vi "Cluster of M and N_UI.vi"(6 "ControlsIndicators":T1, 8 "error in (no error)":errorcluster, 9 "Threshold limits":refnum<vi>, 10 "Index":u8, 11 "Input ListBox Cluster":T7) -> (0 "error out":errorcluster, 3 "ListBox Cluster out":T7)   [LabVIEW 2019, in "ZenGage v3.0 UI.lvclass"]
doc: "This VI checks for entered value Range of connectors, Range for fail, Strict range for connectors and Strict range for fail. If entered values are <1, then it assigns default value 1 to controls."
uses:
  ZenGage v3.0 UI.lvclass
  Type Definitions/Edit tolerance settings/Rack Selection.ctl
  Type Definitions/Edit tolerance settings/Edit Tolerance Input.ctl
  <vilib>/Utility/miscctls.llb/LVPoint32TypeDef.ctl
  Type Definitions/General/Master sample references.ctl
  Type Definitions/Controls and Indicators/Select a part (combobox).ctl
  Type Definitions/Controls and Indicators/EDL control references.ctl
  Type Definitions/Controls and Indicators/Diagnostics control referencs.ctl
  Type Definitions/Controls and Indicators/Inspection control references.ctl
  Type Definitions/Controls and Indicators/General_Control references.ctl
  Type Definitions/Controls and Indicators/Controls and Indicators Cluster.ctl
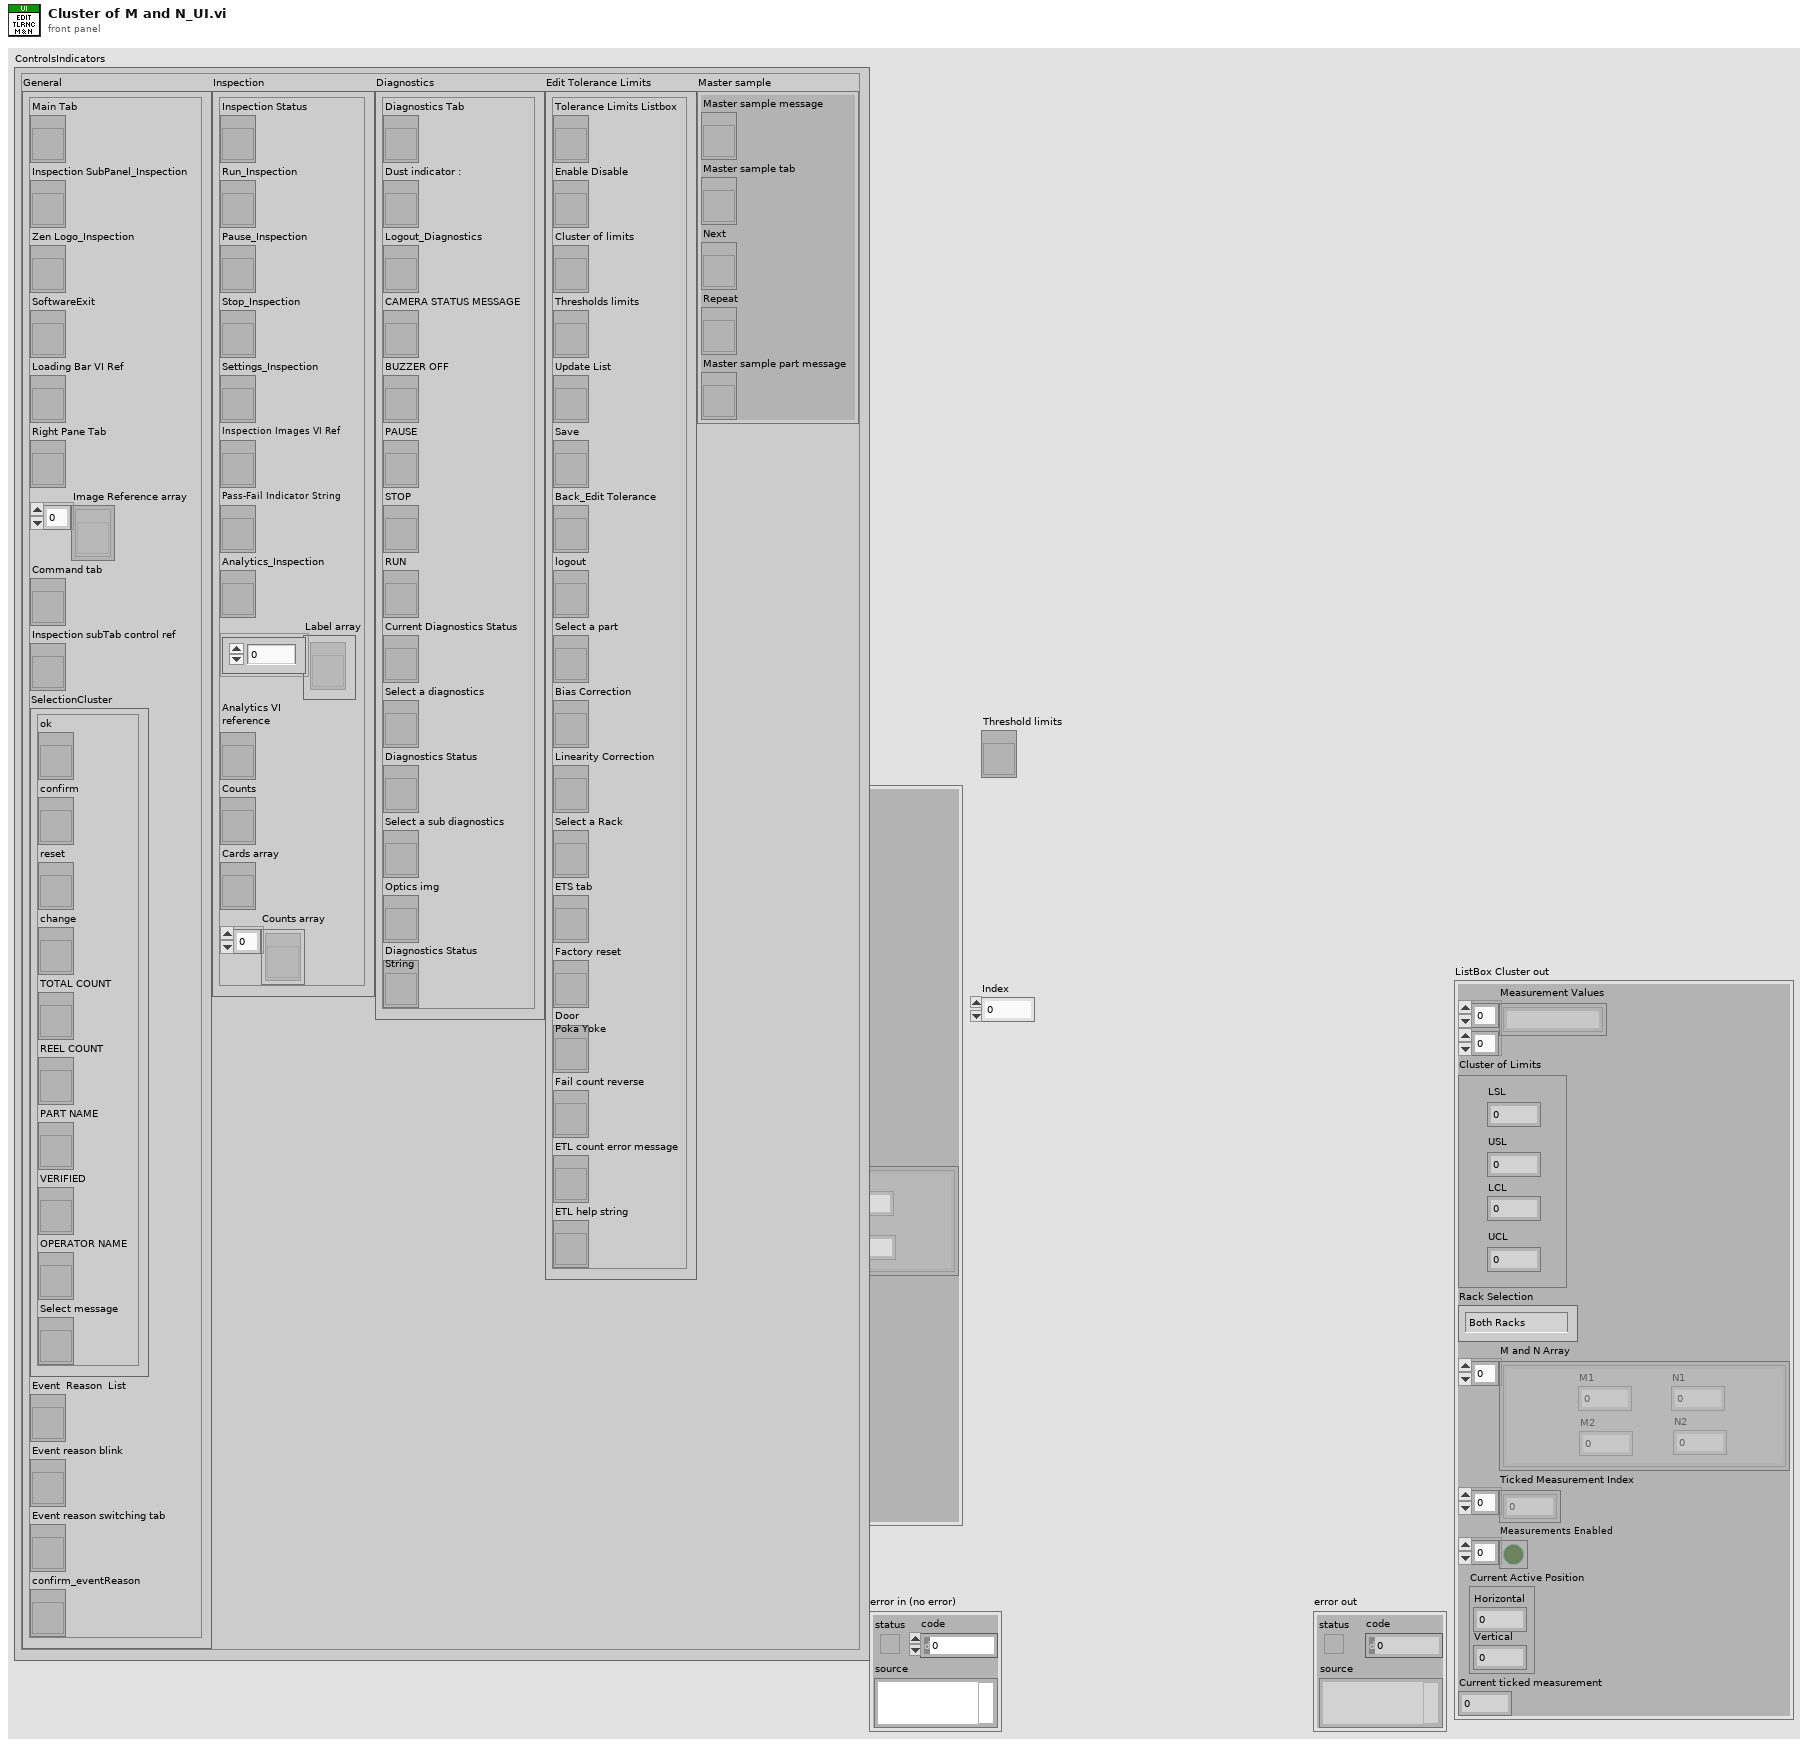
[diagram p1: front panel]
types:
  T1 = typedef "ZenGage v3.0 UI.lvclass/Controls and Indicators Cluster.ctl" = cluster{"General":T2, "Inspection":T3, "Diagnostics":T4, "Edit Tolerance Limits":T5, "Master sample":T6}
  T2 = typedef "ZenGage v3.0 UI.lvclass/General_Control references.ctl" = cluster{"Main Tab":refnum<vi>, "Inspection SubPanel_Inspection":refnum<vi>, "Zen Logo_Inspection":refnum<vi>, "SoftwareExit":refnum<vi>, "Loading Bar VI Ref":refnum<vi>, "Right Pane Tab":refnum<vi>, "Image Reference array":refnum<vi>[], "Command tab":refnum<vi>, "Inspection subTab control ref":refnum<vi>, "SelectionCluster":cluster{"ok":refnum<vi>, "confirm":refnum<vi>, "reset":refnum<vi>, "change":refnum<vi>, "TOTAL COUNT":refnum<vi>, "REEL COUNT":refnum<vi>, "PART NAME":refnum<vi>, "VERIFIED":refnum<vi>, "OPERATOR NAME":refnum<vi>, "Select message":refnum<vi>}, "Event  Reason  List":refnum<vi>, "Event reason blink":refnum<vi>, "Event reason switching tab":refnum<vi>, "confirm_eventReason":refnum<vi>}
  T3 = typedef "ZenGage v3.0 UI.lvclass/Inspection control references.ctl" = cluster{"Inspection Status":refnum<vi>, "Run_Inspection":refnum<vi>, "Pause_Inspection":refnum<vi>, "Stop_Inspection":refnum<vi>, "Settings_Inspection":refnum<vi>, "Inspection Images VI Ref":refnum<vi>, "Pass-Fail Indicator String":refnum<vi>, "Analytics_Inspection":refnum<vi>, "Label array":refnum<vi>[], "Analytics VI\nreference":refnum<vi>, "Counts":refnum<vi>, "Cards array":refnum<vi>, "Counts array":refnum<vi>[]}
  T4 = typedef "ZenGage v3.0 UI.lvclass/Diagnostics control referencs.ctl" = cluster{"Diagnostics Tab":refnum<vi>, "Dust indicator :":refnum<vi>, "Logout_Diagnostics":refnum<vi>, "CAMERA STATUS MESSAGE":refnum<vi>, "BUZZER OFF":refnum<vi>, "PAUSE":refnum<vi>, "STOP":refnum<vi>, "RUN":refnum<vi>, "Current Diagnostics Status":refnum<vi>, "Select a diagnostics":refnum<vi>, "Diagnostics Status":refnum<vi>, "Select a sub diagnostics":refnum<vi>, "Optics img":refnum<vi>, "Diagnostics Status\nString":refnum<vi>}
  T5 = typedef "ZenGage v3.0 UI.lvclass/EDL control references.ctl" = cluster{"Tolerance Limits Listbox":refnum<vi>, "Enable Disable":refnum<vi>, "Cluster of limits":refnum<vi>, "Thresholds limits":refnum<vi>, "Update List":refnum<vi>, "Save":refnum<vi>, "Back_Edit Tolerance":refnum<vi>, "logout":refnum<vi>, "Select a part":refnum<vi>, "Bias Correction":refnum<vi>, "Linearity Correction":refnum<vi>, "Select a Rack":refnum<vi>, "ETS tab":refnum<vi>, "Factory reset":refnum<vi>, "Door\nPoka Yoke":refnum<vi>, "Fail count reverse":refnum<vi>, "ETL count error message":refnum<vi>, "ETL help string":refnum<vi>}
  T6 = typedef "Master sample references.ctl" = cluster{"Master sample message":refnum<vi>, "Master sample tab":refnum<vi>, "Next":refnum<vi>, "Repeat":refnum<vi>, "Master sample part message":refnum<vi>}
  T7 = typedef "ZenGage v3.0 UI.lvclass/Edit Tolerance Input.ctl" = cluster{"Measurement Values":string[][], "Cluster of Limits":cluster{"LSL":dbl, "USL":dbl, "LCL":dbl, "UCL":dbl}, "Rack Selection":T8, "M and N Array":cluster{"M1":u64, "M2":u64, "N1":u64, "N2":u64}[], "Ticked Measurement Index":u32[], "Measurements Enabled":bool[], "Current Active Position":T9, "Current ticked measurement":dbl}
  T8 = typedef "ZenGage v3.0 UI.lvclass/Rack Selection.ctl" = enum16{"Both Racks", "Rack 2", "Rack 1"}
  T9 = typedef "LVPoint32TypeDef.ctl" = cluster{"Horizontal":i32, "Vertical":i32}
  T10 = enum8{"Enabled", "Disabled", "Disabled and Grayed Out"}
  T11 = cluster{"M1":u64, "M2":u64, "N1":u64, "N2":u64}[]
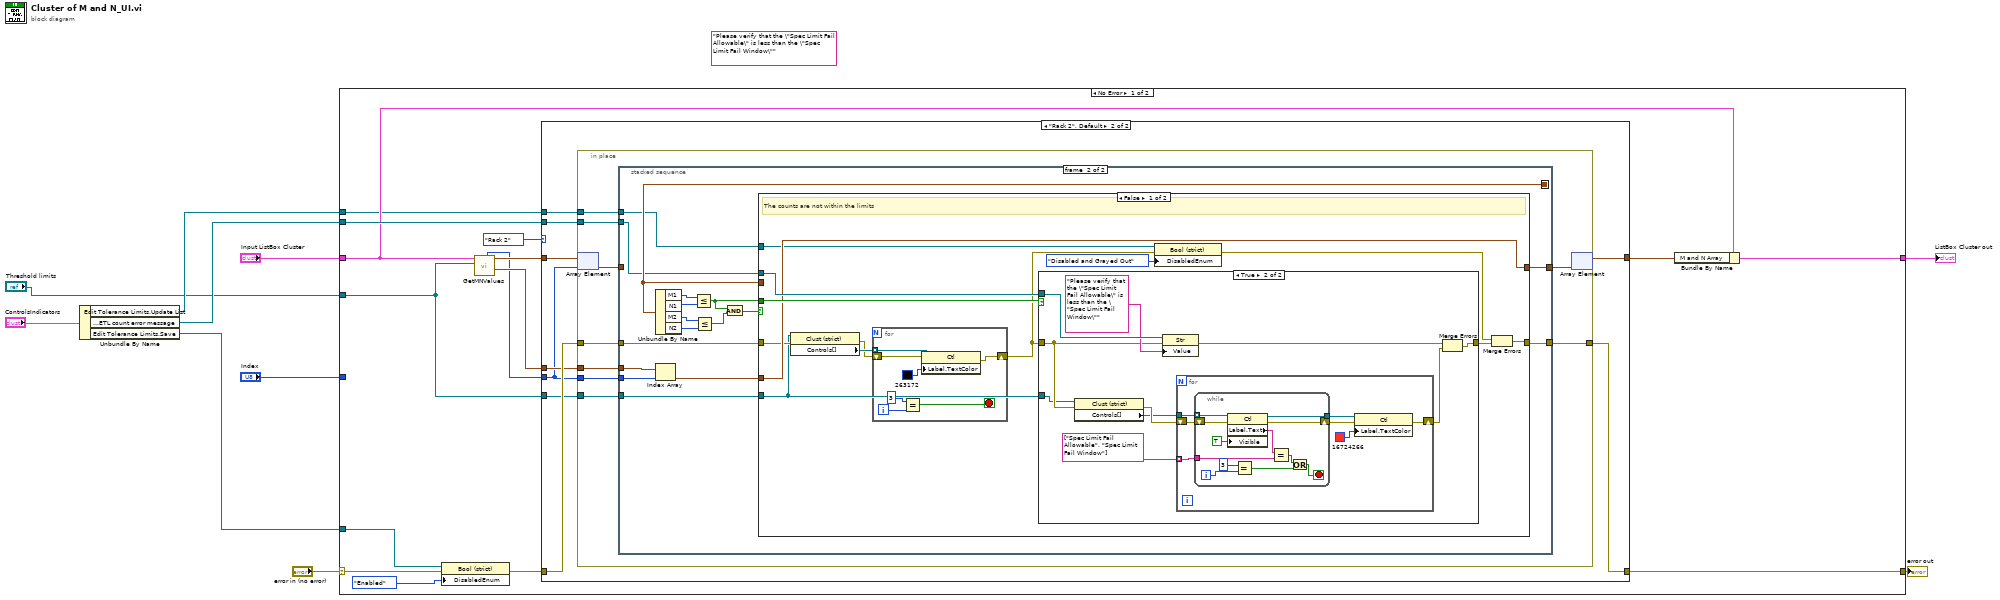
[diagram p0: block diagram]
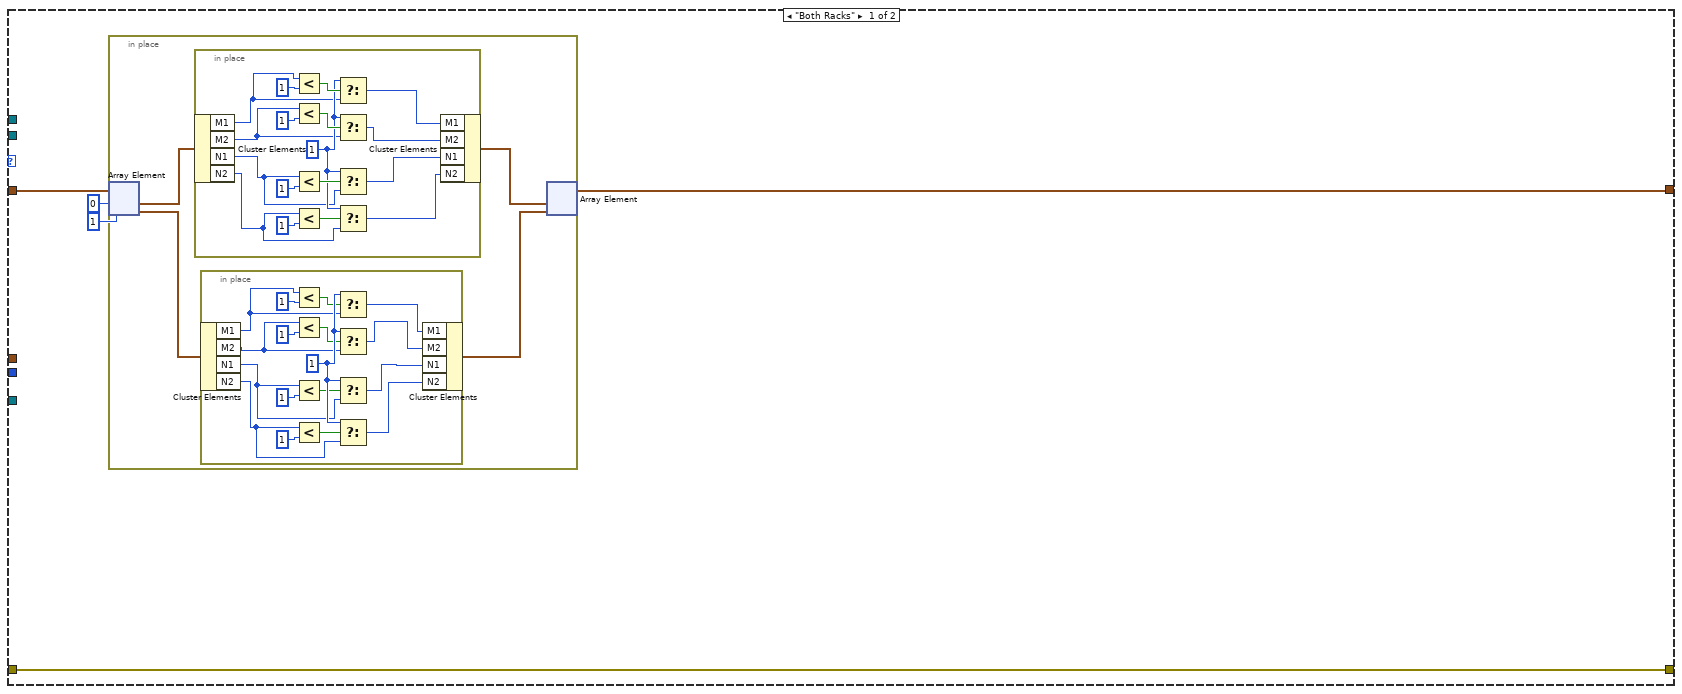
[diagram p2: hidden frame]
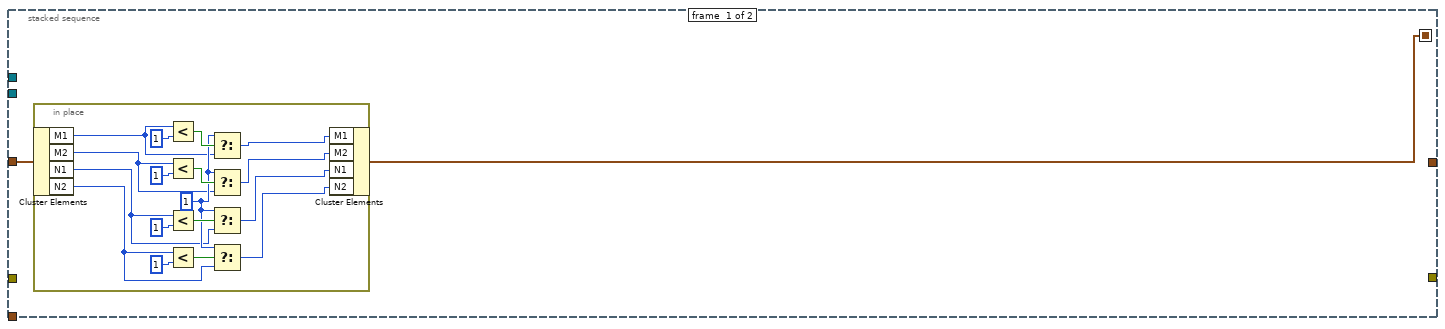
[diagram p3: hidden frame]
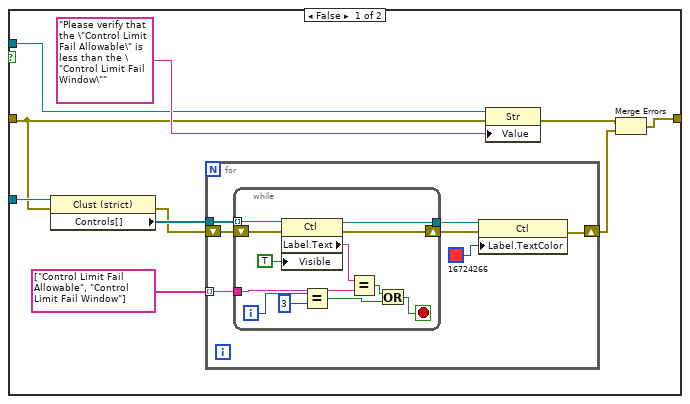
[diagram p4: hidden frame]
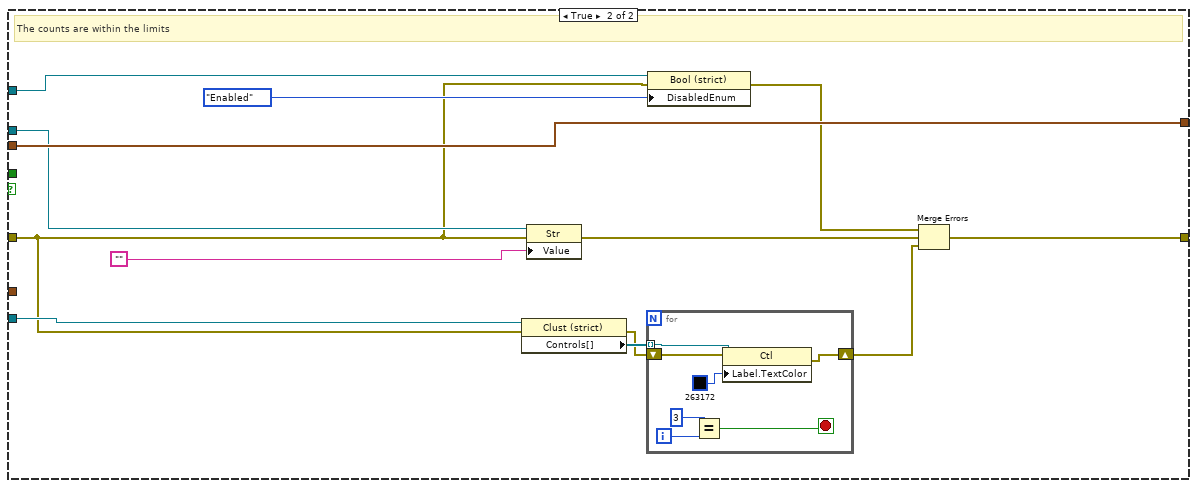
[diagram p5: hidden frame]
diagram:
  (unwired) "Please verify that the \"Spec Limit Fail Allowable\" is less than the \"Spec Limit Fail Window\"" ("Value")
  n1 = Unbundle By Name("ControlsIndicators") -> ("Edit Tolerance Limits.Update List"=w2:refnum<vi>, "Edit Tolerance Limits.ETL count error message"=w4:refnum<vi>, "Edit Tolerance Limits.Save"=w3:refnum<vi>)
  n2 = case shown="No Error" "error in (no error)" {
    selector: "error in (no error)" -> [w18 w222]
    tunnel: [w21 w222] -> w9
    tunnel: [w25 w221] -> w7
    tunnel: "Input ListBox Cluster" -> [w19 w221]
    tunnel: "Index" -> [_ _]
    tunnel: "Threshold limits" -> [w13 _]
    tunnel: w4 -> [w22 _]
    tunnel: w3 -> [w15 _]
    tunnel: w2 -> [w14 _]
    frame No Error {
      n3 = property class="Bool (strict)"(reference=w15, error in=w18, "DisabledEnum"=T10."Enabled" ("Disabled")) -> (error out=w17:errorcluster)  [unwired: 1 out]
      n4 = call "GetMNValues.vi"("Threshold limits"=w13, "Input ListBox Cluster in"=w19) -> ("M and N Array unchanged"=w20:T11, "MN Array changed"=w24:T11, "Last ticked measurement"=w11:u32)  [unwired: 5 in, 2 out]
      n5 = case shown="\"Rack 2\", Default" Rack_Selection."Rack 2" ("Rack Selection") {
        tunnel: w24 -> [w30 w77]
        tunnel: [w27 w76] -> w23
        tunnel: w11 -> [_ w71]
        tunnel: w17 -> [w26 w75]
        tunnel: w22 -> [_ w74]
        tunnel: [w26 w73] -> w21
        tunnel: w20 -> [_ w72]
        tunnel: w13 -> [_ w70]
        tunnel: w14 -> [_ w69]
        frame "Both Racks" {
          n6 = in-place {
            n7 = in-place-array #1(w30, 0, 1) -> (w34:cluster{"M1":u64, "M2":u64, "N1":u64, "N2":u64}, w33:cluster{"M1":u64, "M2":u64, "N1":u64, "N2":u64})
            n8 = in-place {
              w43 = u64 1 ("y")
              n9 = in-place-cluster #2(w34) -> ("M1"=w42:u64, "M2"=w41:u64, "N1"=w40:u64, "N2"=w39:u64)
              n10 = Less?(x=w42, y=u64 1) -> (x < y?=w47:bool)
              n11 = Less?(x=w41, y=u64 1) -> (x < y?=w46:bool)
              n12 = Less?(x=w40, y=u64 1) -> (x < y?=w45:bool)
              n13 = Less?(x=w39, y=u64 1) -> (x < y?=w44:bool)
              n14 = Select(t=w43, s=w47, f=w42) -> (s? t:f=w38:u64)
              n15 = Select(t=w43, s=w46, f=w41) -> (s? t:f=w37:u64)
              n16 = Select(t=w43, s=w45, f=w40) -> (s? t:f=w36:u64)
              n17 = Select(t=w43, s=w44, f=w39) -> (s? t:f=w35:u64)
              n18 = in-place-cluster #2("M1"=w38, "M2"=w37, "N1"=w36, "N2"=w35) -> (w31:cluster{"M1":u64, "M2":u64, "N1":u64, "N2":u64})
            }
            n19 = in-place {
              w68 = u64 1 ("y")
              n20 = in-place-cluster #3(w33) -> ("M1"=w59:u64, "M2"=w58:u64, "N1"=w57:u64, "N2"=w56:u64)
              n21 = Less?(x=w59, y=u64 1) -> (x < y?=w64:bool)
              n22 = Less?(x=w58, y=u64 1) -> (x < y?=w65:bool)
              n23 = Less?(x=w57, y=u64 1) -> (x < y?=w66:bool)
              n24 = Less?(x=w56, y=u64 1) -> (x < y?=w67:bool)
              n25 = Select(t=w68, s=w64, f=w59) -> (s? t:f=w55:u64)
              n26 = Select(t=w68, s=w65, f=w58) -> (s? t:f=w54:u64)
              n27 = Select(t=w68, s=w66, f=w57) -> (s? t:f=w53:u64)
              n28 = Select(t=w68, s=w67, f=w56) -> (s? t:f=w52:u64)
              n29 = in-place-cluster #3("M1"=w55, "M2"=w54, "N1"=w53, "N2"=w52) -> (w32:cluster{"M1":u64, "M2":u64, "N1":u64, "N2":u64})
            }
            n30 = in-place-array #1(w31, w32) -> (w27:T11)  [unwired: 2 out]
          }
        }
        frame "Rack 2", Default {
          n31 = in-place {
            in-place-border: w75 -> [w84]
            in-place-border: w74 -> [w83]
            in-place-border: [w82] -> w73
            in-place-border: w72 -> [w81]
            in-place-border: w71 -> [w80]
            in-place-border: w70 -> [w79]
            in-place-border: w69 -> [w78]
            n32 = in-place-array #4(w77, w71) -> (w86:cluster{"M1":u64, "M2":u64, "N1":u64, "N2":u64})
            n33 = stacked-sequence {
              seq-local: [w87 _] -> [_ w116]
              tunnel: w86 -> [w88 _]
              tunnel: [_ w115] -> w85
              tunnel: w84 -> [_ w113]
              tunnel: w83 -> [_ w112]
              tunnel: [_ w111] -> w82
              tunnel: w81 -> [_ w110]
              tunnel: w80 -> [_ w109]
              tunnel: w79 -> [_ w107]
              tunnel: w78 -> [_ w106]
              frame #0 {
                n34 = in-place {
                  w97 = u64 1 ("y")
                  n35 = in-place-cluster #5(w88) -> ("M1"=w96:u64, "M2"=w95:u64, "N1"=w94:u64, "N2"=w93:u64)
                  n36 = Less?(x=w96, y=u64 1) -> (x < y?=w101:bool)
                  n37 = Less?(x=w95, y=u64 1) -> (x < y?=w100:bool)
                  n38 = Less?(x=w94, y=u64 1) -> (x < y?=w99:bool)
                  n39 = Less?(x=w93, y=u64 1) -> (x < y?=w98:bool)
                  n40 = Select(t=w97, s=w101, f=w96) -> (s? t:f=w92:u64)
                  n41 = Select(t=w97, s=w100, f=w95) -> (s? t:f=w91:u64)
                  n42 = Select(t=w97, s=w99, f=w94) -> (s? t:f=w90:u64)
                  n43 = Select(t=w97, s=w98, f=w93) -> (s? t:f=w89:u64)
                  n44 = in-place-cluster #5("M1"=w92, "M2"=w91, "N1"=w90, "N2"=w89) -> (w87:cluster{"M1":u64, "M2":u64, "N1":u64, "N2":u64})
                }
              }
              frame #1 {
                n45 = Unbundle By Name(w116) -> ("M1"=w122:u64, "N1"=w121:u64, "M2"=w120:u64, "N2"=w119:u64)
                n46 = Index Array(array=w110, index=w109) -> (element=w108:cluster{"M1":u64, "M2":u64, "N1":u64, "N2":u64})
                n47 = Less Or Equal?(x=w122, y=w121) -> (x <= y?=w114:bool)
                n48 = Less Or Equal?(x=w120, y=w119) -> (x <= y?=w118:bool)
                n49 = And(x=w114, y=w118) -> (x .and. y?=w117:bool)
                n50 = case shown="False" w117 {
                  tunnel: w116 -> [_ w213]
                  tunnel: [w133 w213] -> w115
                  tunnel: w114 -> [w135 _]
                  tunnel: w113 -> [w125 w203]
                  tunnel: w112 -> [w134 w209]
                  tunnel: [w129 w206] -> w111
                  tunnel: w108 -> [w133 _]
                  tunnel: w107 -> [w124 w212]
                  tunnel: w106 -> [w132 w202]
                  frame False {
                    # "The counts are not within the limits"
                    n51 = property class="Clust (strict)"(reference=w124, error in=w125) -> (error out=w126:errorcluster, "Controls[]"=w127:refnum<vi>[])  [unwired: 1 out]
                    n52 = for {
                      tunnel: w127 -> [w140] mode=indexing
                      shift-right: [w139] -> w123
                      shift-left: w126 -> [w141]
                      i -> [w138]
                      stop <- w136 stop-if-true
                      n53 = Equal?(x=3, y=w138) -> (x = y?=w136:bool)
                      n54 = property class="Ctl"(reference=w140, error in=w141, "Label.TextColor"=u32 263172) -> (error out=w139:errorcluster)  [unwired: 1 out]
                    }
                    n55 = case shown="True" w135 {
                      tunnel: w123 -> [w149 w176]
                      tunnel: w134 -> [w151 w181]
                      tunnel: [w143 w172] -> w130
                      tunnel: w124 -> [w150 w175]
                      frame False {
                        n56 = property class="Clust (strict)"(reference=w150, error in=w149) -> (error out=w147:errorcluster, "Controls[]"=w148:refnum<vi>[])  [unwired: 1 out]
                        n57 = for {
                          tunnel: w148 -> [w159]
                          shift-right: [w155] -> w145
                          shift-left: w147 -> [w158]
                          tunnel: string[] ["Control Limit Fail Allowable", "Control Limit Fail Window"] -> [w157] mode=indexing
                          n58 = while {
                            tunnel: w159 -> [w171] mode=indexing
                            shift-right: [w169] -> w156
                            shift-left: w158 -> [w170]
                            tunnel: w157 -> [w167]
                            tunnel: [w166] -> w154
                            i -> [w163]
                            stop <- w161 stop-if-true
                            n59 = property class="Ctl"(reference=w171, error in=w170, "Visible"=TRUE) -> (reference out=w166:refnum<vi>, error out=w169:errorcluster, "Label.Text"=w168:string)
                            n60 = Equal?(x=w163, y=3) -> (x = y?=w164:bool)
                            n61 = Equal?(x=w168, y=w167) -> (x = y?=w165:bool)
                            n62 = Or(x=w165, y=w164) -> (x .or. y?=w161:bool)
                          }
                          n63 = property class="Ctl"(reference=w154, error in=w156, "Label.TextColor"=u32 16724266) -> (error out=w155:errorcluster)  [unwired: 1 out]
                        }
                        n64 = property class="Str"(reference=w151, error in=w149, "Value"="Please verify that the \"Control Limit Fail Allowable\" is less than the \"Control Limit Fail Window\"") -> (error out=w144:errorcluster)  [unwired: 1 out]
                        n65 = Merge Errors(w144, w145) -> (w143:errorcluster)
                      }
                      frame True {
                        n66 = property class="Clust (strict)"(reference=w175, error in=w176) -> (error out=w178:errorcluster, "Controls[]"=w177:refnum<vi>[])  [unwired: 1 out]
                        n67 = property class="Str"(reference=w181, error in=w176, "Value"="Please verify that the \"Spec Limit Fail Allowable\" is less than the \"Spec Limit Fail Window\"") -> (error out=w174:errorcluster)  [unwired: 1 out]
                        n68 = for {
                          tunnel: w177 -> [w188]
                          shift-right: [w184] -> w173
                          shift-left: w178 -> [w187]
                          tunnel: string[] ["Spec Limit Fail Allowable", "Spec Limit Fail Window"] -> [w186] mode=indexing
                          n69 = while {
                            tunnel: w188 -> [w200] mode=indexing
                            shift-right: [w198] -> w185
                            shift-left: w187 -> [w199]
                            tunnel: w186 -> [w196]
                            tunnel: [w195] -> w183
                            i -> [w194]
                            stop <- w190 stop-if-true
                            n70 = property class="Ctl"(reference=w200, error in=w199, "Visible"=TRUE) -> (reference out=w195:refnum<vi>, error out=w198:errorcluster, "Label.Text"=w197:string)
                            n71 = Equal?(x=3, y=w194) -> (x = y?=w192:bool)
                            n72 = Equal?(x=w197, y=w196) -> (x = y?=w191:bool)
                            n73 = Or(x=w191, y=w192) -> (x .or. y?=w190:bool)
                          }
                          n74 = property class="Ctl"(reference=w183, error in=w185, "Label.TextColor"=u32 16724266) -> (error out=w184:errorcluster)  [unwired: 1 out]
                        }
                        n75 = Merge Errors(w174, w173) -> (w172:errorcluster)
                      }
                    }
                    n76 = property class="Bool (strict)"(reference=w132, error in=w123, "DisabledEnum"=T10."Disabled and Grayed Out" ("Disabled")) -> (error out=w128:errorcluster)  [unwired: 1 out]
                    n77 = Merge Errors(w128, w130) -> (w129:errorcluster)
                  }
                  frame True {
                    # "The counts are within the limits"
                    n78 = property class="Clust (strict)"(reference=w212, error in=w203) -> (error out=w210:errorcluster, "Controls[]"=w211:refnum<vi>[])  [unwired: 1 out]
                    n79 = property class="Str"(reference=w209, error in=w203, "Value"="") -> (error out=w208:errorcluster)  [unwired: 1 out]
                    n80 = for {
                      tunnel: w211 -> [w218] mode=indexing
                      shift-right: [w217] -> w207
                      shift-left: w210 -> [w219]
                      i -> [w216]
                      stop <- w214 stop-if-true
                      n81 = Equal?(x=3, y=w216) -> (x = y?=w214:bool)
                      n82 = property class="Ctl"(reference=w218, error in=w219, "Label.TextColor"=u32 263172) -> (error out=w217:errorcluster)  [unwired: 1 out]
                    }
                    n83 = property class="Bool (strict)"(reference=w202, error in=w203, "DisabledEnum"=T10."Enabled" ("Disabled")) -> (error out=w201:errorcluster)  [unwired: 1 out]
                    n84 = Merge Errors(w201, w208, w207) -> (w206:errorcluster)
                  }
                }
              }
            }
            n85 = in-place-array #4(w85) -> (w76:T11)  [unwired: 1 out]
          }
        }
      }
      n86 = Bundle By Name(cluster=w19, "M and N Array"=w23) -> (w25:T7)
    }
    frame Error {
    }
  }
  "error out" <- w9
  "ListBox Cluster out" <- w7
